vi "Set FIFO.vi"(10 "FIFO":refnum<k33>, 11 "Pool in":refnum<class "Pool.lvclass">) -> (3 "Pool out":refnum<class "Pool.lvclass">)   [LabVIEW 2017, in "DSF Core.lvlib" / "Pool.lvclass"]
uses:
  Pool.lvclass
  Pool.lvclass/Pool.ctl
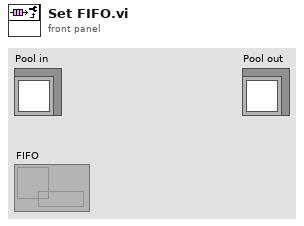
[diagram p1: front panel]
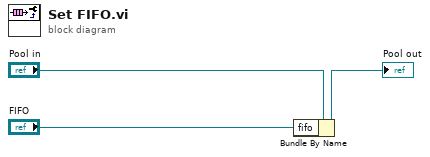
[diagram p0: block diagram]
diagram:
  n1 = Bundle By Name(cluster="Pool in", "fifo"="FIFO") -> (→"Pool out":refnum<class "Pool.lvclass">)
